vi "List Bucket Contents.vi"(8 "error in (no error)":errorcluster, 11 "Data.S3":refnum<class "Data.S3.lvclass">) -> (0 "error out":errorcluster, 1 "Common Prefixes":string[](array[string]), 2 "Objects in bucket":T1[](array[typedef]), 3 "Data.S3 out":refnum<class "Data.S3.lvclass">)   [LabVIEW 2020, in "Data.S3.lvclass"]
uses:
  Data.S3.lvclass
  <vilib>/AWS Toolkit/S3/Object Content.ctl
  <vilib>/AWS Toolkit/S3/Storage Class.ctl
  <vilib>/AWS Toolkit/S3/Owner.ctl
  Data.S3.lvclass/Data.S3.ctl
  <vilib>/AWS Toolkit/S3/Bucket/Bucket.lvclass
  <vilib>/AWS Toolkit/S3/NI_AWS_S3.lvlib
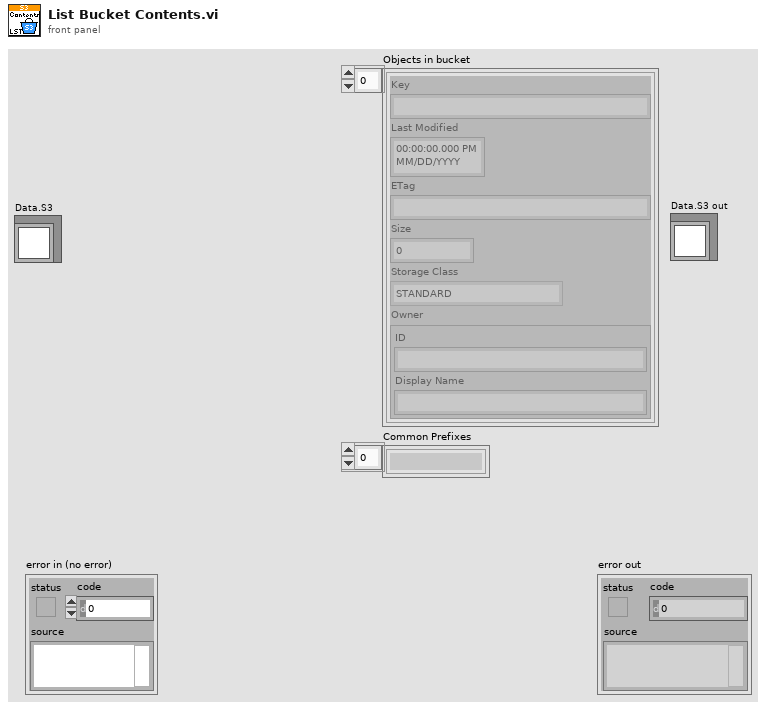
[diagram p1: front panel]
types:
  T1 = typedef "NI_AWS_S3.lvlib/Object Content.ctl" = cluster{"Key":string, "Last Modified":timestamp, "ETag":string, "Size":u64, "Storage Class":T2, "Owner":T3}
  T2 = typedef "NI_AWS_S3.lvlib/Storage Class.ctl" = enum16{"STANDARD", "REDUCED_REDUNDANCY"}
  T3 = typedef "NI_AWS_S3.lvlib/Owner.ctl" = cluster{"ID":string, "Display Name":string}
  T4 = typedef "NI_AWS_Core.lvlib/HTTP Request.lvclass/AWS Credentials.ctl" = cluster{"Access Key":string, "Secret Key":string}
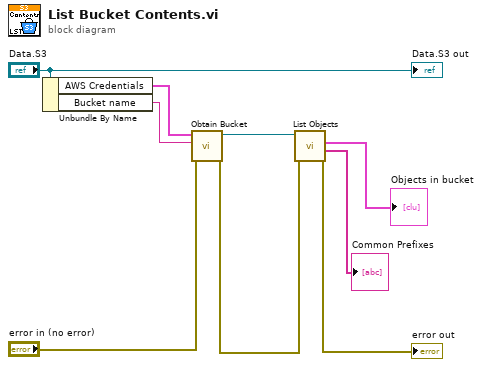
[diagram p0: block diagram]
diagram:
  n1 = Unbundle By Name("Data.S3") -> ("AWS Credentials"=w5:T4, "Bucket name"=w4:string)
  n2 = call <vilib>:"Obtain Bucket.vi"("error in (no error)"="error in (no error)", "Bucket name"=w4, "AWS Credentials"=w5) -> ("error out"=w8:errorcluster, "Bucket"=w6:refnum<class "Bucket.lvclass">)  [unwired: 7 in]
  n3 = call <vilib>:"List Objects.vi"("error in (no error)"=w8, "Bucket in"=w6) -> ("error out"=→"error out":errorcluster, "Common Prefixes"=→"Common Prefixes":string[], "Objects"=→"Objects in bucket":T1[])  [unwired: 6 in, 1 out]
  "Data.S3 out" <- "Data.S3"
